vi "Smart Buffer (DBL) 2.vi"(8 "destructive reads (yes:T)":bool=TRUE, 10 "new element [write]":dbl format="%0.2f", 11 "mode":T1(ring)) -> (0 "number unread after":i32, 1 "entire buffer [read all]":dbl[](array[numeric]) format="%0.2f", 2 "oldest/newest element [read one]":dbl format="%0.2f", 3 "output valid? [read]":bool, 4 "buffer size":i32, 5 "number written after":u32)   [LabVIEW 2012]
doc: "This \"smart\" buffer works like a queue or FIFO (first-in, first-out) buffer or like a stack or LIFO (last-in, first-out) buffer or like a write-one-at-a-time, read-all buffer, and its size adjusts automatically in stages as it fills. In addition, you can read the the data once (destructively) or many times (nondestructively). The VI is non-reentrant and acts like a global variable; use a copy of it under a different name for each buffer in your program. \n\nThe modes are empty (0), write (1), read oldest (2), read newest (3), and read all (4). See the front panel instructions for more information."
panel:
  # "Execute with mode set to empty before you start and after you finish; this sets the buffer size to zero.  As you write elements, the buffer expands first to 16 elements, and when it fills that space, expands by doubling in size until it reaches 512 elements, then expands by units of 512 elements.  It contracts only when you empty it.  Number written after is the total number of points written to date after the call finishes.  \n\nTo operate the buffer like a queue or FIFO, set the mode to read oldest.  To operate it like a stack of LIFO, set the mode to read newest.  To read the entire buffer, set the mode to read all.  If destructive reads is TRUE (default), these operations adjust the buffer pointers and the number unread after and you cannot read the same data twice.  With nondestructive reads, you can read the data multiple times.  output valid? is TRUE if the buffer is not empty on reads.\n\nTo change the data type from DBL, simply replace the controls new element, oldest/newest element, and the DBL in entire buffer with a scalar of the desired type.  If you want the data type to be an array or a set of elements, put them into a cluster."
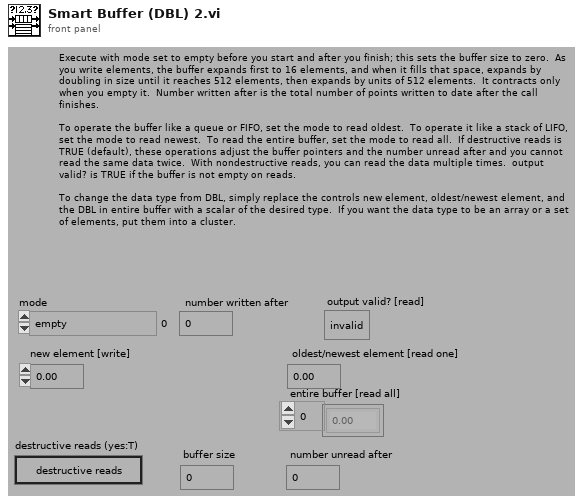
[diagram p1: front panel]
types:
  T1 = enum16{"empty", "write", "read oldest (queue)", "read newest (stack)", "read all"}
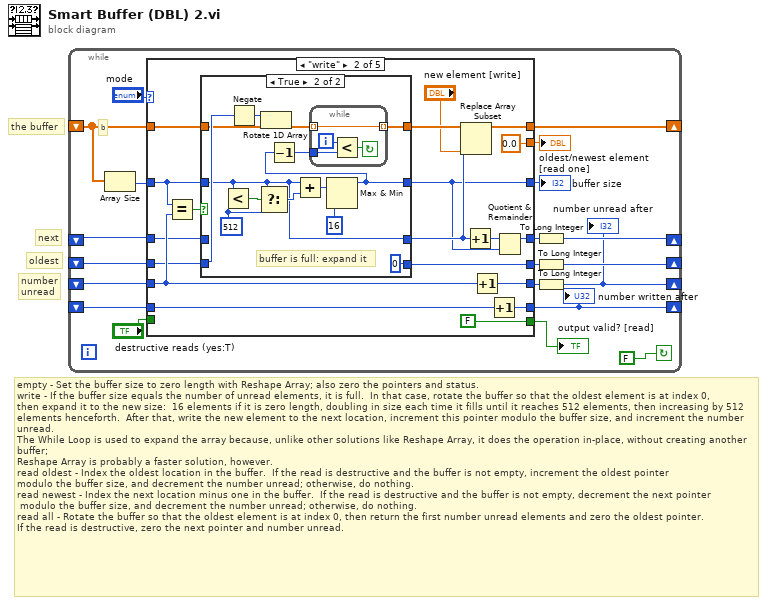
[diagram p0: block diagram]
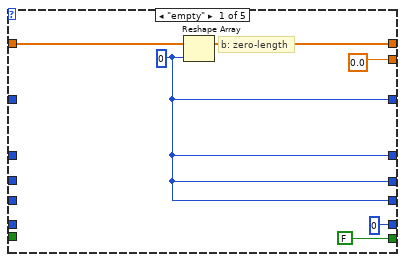
[diagram p2: hidden frame]
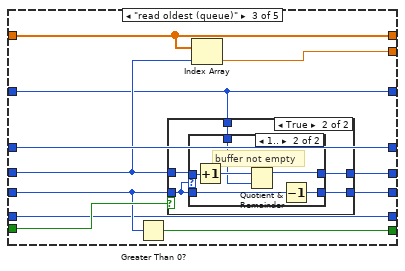
[diagram p4: hidden frame]
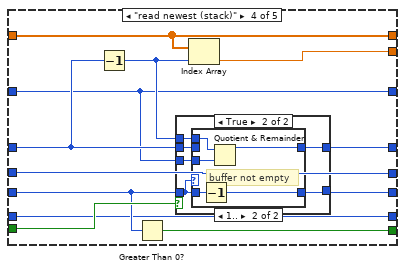
[diagram p7: hidden frame]
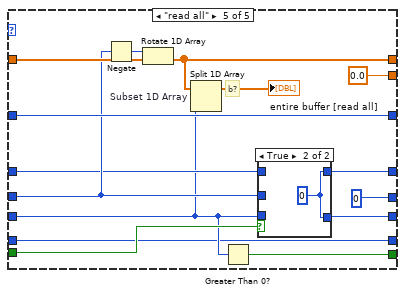
[diagram p10: hidden frame]
diagram:
  # "the buffer"
  # "number unread"
  # "oldest"
  # "next"
  # "empty - Set the buffer size to zero length with Reshape Array; also zero the pointers and status.\nwrite - If the buffer size equals the number of unread elements, it is full.  In that case, rotate the buffer so that the oldest element is at index 0, \nthen expand it to the new size:  16 elements if it is zero length, doubling in size each time it fills until it reaches 512 elements, then increasing by 512 \nelements henceforth.  After that, write the new element to the next location, increment this pointer modulo the buffer size, and increment the number unread.  \nThe While Loop is used to expand the array because, unlike other solutions like Reshape Array, it does the operation in-place, without creating another buffer; \nReshape Array is probably a faster solution, however.\nread oldest - Index the oldest location in the buffer.  If the read is destructive and the buffer is not empty, increment the oldest pointer \nmodulo the buffer size, and decrement the number unread; otherwise, do nothing.\nread newest - Index the next location minus one in the buffer.  If the read is destructive and the buffer is not empty, decrement the next pointer\n modulo the buffer size, and decrement the number unread; otherwise, do nothing.\nread all - Rotate the buffer so that the oldest element is at index 0, then return the first number unread elements and zero the oldest pointer.  \nIf the read is destructive, zero the next pointer and number unread."
  n1 = while {
    shift-left: _ -> [w3]
    shift-right: [w1] -> _
    shift-left: _ -> [w19]
    shift-right: [w4] -> _
    shift-left: _ -> [w14]
    shift-right: [w5] -> _
    shift-left: _ -> [w11]
    shift-right: [w20] -> _
    shift-left: _ -> [w13]
    shift-right: [w6] -> _
    stop <- FALSE continue-if-true
    # "b"
    n2 = Array Size(array=w11) -> (size(s)=w12:i32)
    n3 = case shown="\"write\"" "mode" {
      tunnel: [w23 w30 w77 w99 w128] -> w17
      tunnel: w13 -> [_ w35 w77 w98 w125]
      tunnel: [w25 w45 w78 w105 w133] -> w20
      tunnel: w11 -> [w26 w37 w78 w105 w134]
      tunnel: w14 -> [_ w36 w72 w102 w126]
      tunnel: [w23 w42 w75 w102 0] -> w18
      tunnel: [w23 w44 w74 w95 w127] -> w7
      tunnel: w19 -> [_ w41 w70 w100 w122]
      tunnel: [FALSE FALSE w69 w103 w132] -> w16
      tunnel: w12 -> [_ w39 w71 w96 w130]
      tunnel: [w23 w31 w71 w96 w130] -> w10
      tunnel: [0.0 0.0 w76 w104 0.0] -> w9
      tunnel: "destructive reads (yes:T)" -> [_ _ w73 w101 w124]
      tunnel: w3 -> [_ w28 w68 w94 w121]
      tunnel: [u32 0 w27 w68 w94 w121] -> w1
      frame "empty" {
        w23 = 0
        # "b: zero-length"
        n4 = Reshape Array "Reshape Array"(w26, w23) -> (w25:dbl[])
      }
      frame "write" {
        n5 = Equal?(x=w39, y=w41) -> (x = y?=w40:bool)
        n6 = case shown="True" w40 {
          tunnel: [w46 w55] -> w33
          tunnel: [w48 w53] -> w31
          tunnel: [w47 0] -> w42
          tunnel: w36 -> [w47 w61]
          tunnel: [w49 w50] -> w38
          tunnel: w39 -> [w48 w55]
          tunnel: w37 -> [w49 w54]
          tunnel: w35 -> [w46 _]
          frame False {
          }
          frame True {
            w58 = 512
            # "buffer is full: expand it"
            n7 = Less?(x=w55, y=w58) -> (x < y?=w60:bool)
            n8 = Negate(x=w61) -> (-x=w62:i32)
            n9 = Select(t=w55, s=w60, f=w58) -> (s? t:f=w59:i32)
            n10 = Rotate 1D Array(1:w54, 2:w62) -> (0:w51:dbl[])
            n11 = Add(x=w55, y=w59) -> (x+y=w57:i32)
            n12 = Max & Min(x=w57, y=16) -> (max(x,y)=w53:i32)  [unwired: 1 out]
            n13 = Decrement(x=w53) -> (x-1=w52:i32)
            n14 = while {
              tunnel: [w64] -> w50 mode=indexing
              tunnel: w51 -> [w64] mode=indexing
              tunnel: w52 -> [w67]
              i -> [w66]
              stop <- w65 continue-if-true
              n15 = Less?(x=w66, y=w67) -> (x < y?=w65:bool)
            }
          }
        }
        n16 = Replace Array Subset(array=w38, new element="new element [write]", index=w33) -> (w45:dbl[])
        n17 = Increment(x=w33) -> (x+1=w32:i32)
        n18 = Increment(x=w41) -> (x+1=w44:i32)
        n19 = Increment(x=w28) -> (x+1=w27:u32)
        n20 = Quotient & Remainder(x=w32, y=w31) -> (x-y*floor(x/y)=w30:i32)  [unwired: 1 out]
      }
      frame "read oldest (queue)" {
        n21 = Greater Than 0?(x=w70) -> (x > 0?=w69:bool)
        n22 = case shown="True" w73 {
          tunnel: w70 -> [w79 w83]
          tunnel: w72 -> [w80 w85]
          tunnel: [w80 w82] -> w75
          tunnel: [w79 w84] -> w74
          tunnel: w71 -> [_ w81]
          frame False {
          }
          frame True {
            n23 = case shown="1.." w83 {
              tunnel: w83 -> [w87 w93]
              tunnel: [w87 w92] -> w84
              tunnel: w85 -> [w86 w91]
              tunnel: [w86 w89] -> w82
              tunnel: w81 -> [_ w88]
              frame ..0 {
                # "buffer empty"
              }
              frame 1.. {
                # "buffer not empty"
                n24 = Increment(x=w91) -> (x+1=w90:i32)
                n25 = Quotient & Remainder(x=w90, y=w88) -> (x-y*floor(x/y)=w89:i32)  [unwired: 1 out]
                n26 = Decrement(x=w93) -> (x-1=w92:i32)
              }
            }
          }
        }
        n27 = Index Array(array=w78, index=w72) -> (element=w76:dbl)
      }
      frame "read newest (stack)" {
        n28 = Decrement(x=w98) -> (x-1=w97:i32)
        n29 = Greater Than 0?(x=w100) -> (x > 0?=w103:bool)
        n30 = case shown="True" w101 {
          tunnel: w100 -> [w107 w113]
          tunnel: [w107 w112] -> w95
          tunnel: [w106 w109] -> w99
          tunnel: w98 -> [w106 w108]
          tunnel: w97 -> [_ w110]
          tunnel: w96 -> [_ w111]
          frame False {
          }
          frame True {
            n31 = case shown="1.." w113 {
              tunnel: w113 -> [w115 w120]
              tunnel: [w115 w119] -> w112
              tunnel: w111 -> [_ w118]
              tunnel: w110 -> [_ w117]
              tunnel: [w114 w116] -> w109
              tunnel: w108 -> [w114 _]
              frame ..0 {
                # "buffer empty"
              }
              frame 1.. {
                # "buffer not empty"
                n32 = Decrement(x=w120) -> (x-1=w119:i32)
                n33 = Quotient & Remainder(x=w117, y=w118) -> (x-y*floor(x/y)=w116:i32)  [unwired: 1 out]
              }
            }
          }
        }
        n34 = Index Array "Index Array"(array=w105, index=w97) -> (element=w104:dbl)
      }
      frame "read all" {
        # "b?"
        n35 = Negate(x=w126) -> (-x=w135:i32)
        n36 = Rotate 1D Array(1:w134, 2:w135) -> (0:w133:dbl[])
        n37 = Split 1D Array "Subset 1D Array"(array=w133, index=w122) -> (first subarray=→"entire buffer [read all]":dbl[])  [unwired: 1 out]
        n38 = Greater Than 0?(x=w122) -> (x > 0?=w132:bool)
        n39 = case shown="True" w124 {
          tunnel: [w136 w137] -> w128
          tunnel: [w136 w137] -> w127
          tunnel: w122 -> [w136 _]
          tunnel: w126 -> [_ _]
          tunnel: w125 -> [_ _]
          frame False {
          }
          frame True {
            w137 = 0
          }
        }
      }
    }
    "output valid? [read]" <- w16
    "buffer size" <- w10
    "oldest/newest element [read one]" <- w9
    "number written after" <- w1
    n40 = To Long Integer(number=w17) -> (32bit integer=w6:i32)
    n41 = To Long Integer(number=w18) -> (32bit integer=w5:i32)
    n42 = To Long Integer(number=w7) -> (32bit integer=w4:i32)
    "number unread after" <- w4
  }
